vi "user32.FindWindow.vi"(8 "error in":errorcluster caption="error in (no error)", 9 "Window Title":string) -> (0 "error out":errorcluster, 1 "hWnd":u32)   [LabVIEW 2018]
uses:
  User32.dll
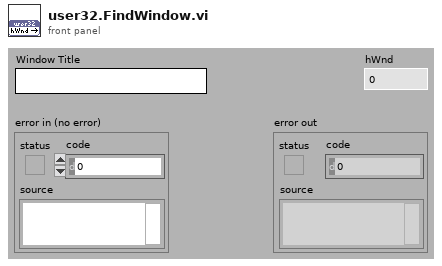
[diagram p1: front panel]
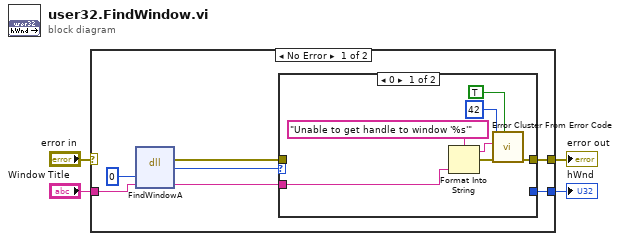
[diagram p0: block diagram]
diagram:
  n1 = case shown="No Error" "error in" {
    selector: "error in" -> [_ w21]
    tunnel: [w8 w21] -> w3
    tunnel: [w7 _] -> w2
    tunnel: "Window Title" -> [w6 _]
    frame No Error {
      n2 = dll-call lib="User32.dll" fn="FindWindowA"("lpszClassName"=u32 0, "lpszWindowName"=w6) -> (error out=w9:errorcluster, "hWnd"=w10:u32, "lpszWindowName"=w5:string)  [unwired: 4 in, 1 out]
      n3 = case shown="0" w10 {
        selector: w10 -> [_ w19]
        tunnel: w9 -> [_ w20]
        tunnel: [w16 w20] -> w8
        tunnel: w5 -> [w18 _]
        tunnel: [_ w19] -> w7
        frame 0 {
          n4 = Format Into String(format string="Unable to get handle to window '%s'", w18) -> (resulting string=w14:string, error out=w15:errorcluster)  [unwired: 2 in]
          n5 = call <vilib>:"Error Cluster From Error Code.vi"("show call chain? (False)"=TRUE, "error in (no error)"=w15, "error message (\"\")"=w14, "error code (0)"=42) -> ("error out"=w16:errorcluster)  [unwired: 5 in]
        }
        frame Default {
        }
      }
    }
    frame Error {
    }
  }
  "error out" <- w3
  "hWnd" <- w2
